vi "Main_No_OOP.vi"() -> ()   [LabVIEW 2020]
uses:
  <vilib>/vision/driver/NI_Vision_Acquisition_Software.lvlib
panel:
  in  "Stop":bool
  in  "Tipo de Cámara":enum32{"WebCam", "Simulada"}(tab)
  in  "Camaras Disponibles":u16(ring) items=["cam0", "cam1", "cam2", "cam3", "cam4"]
  in  "Aceptar":bool
  in  "Ruta IMG":path
  in  "Aceptar":bool
  out "Imagen":T1(plugin-control)
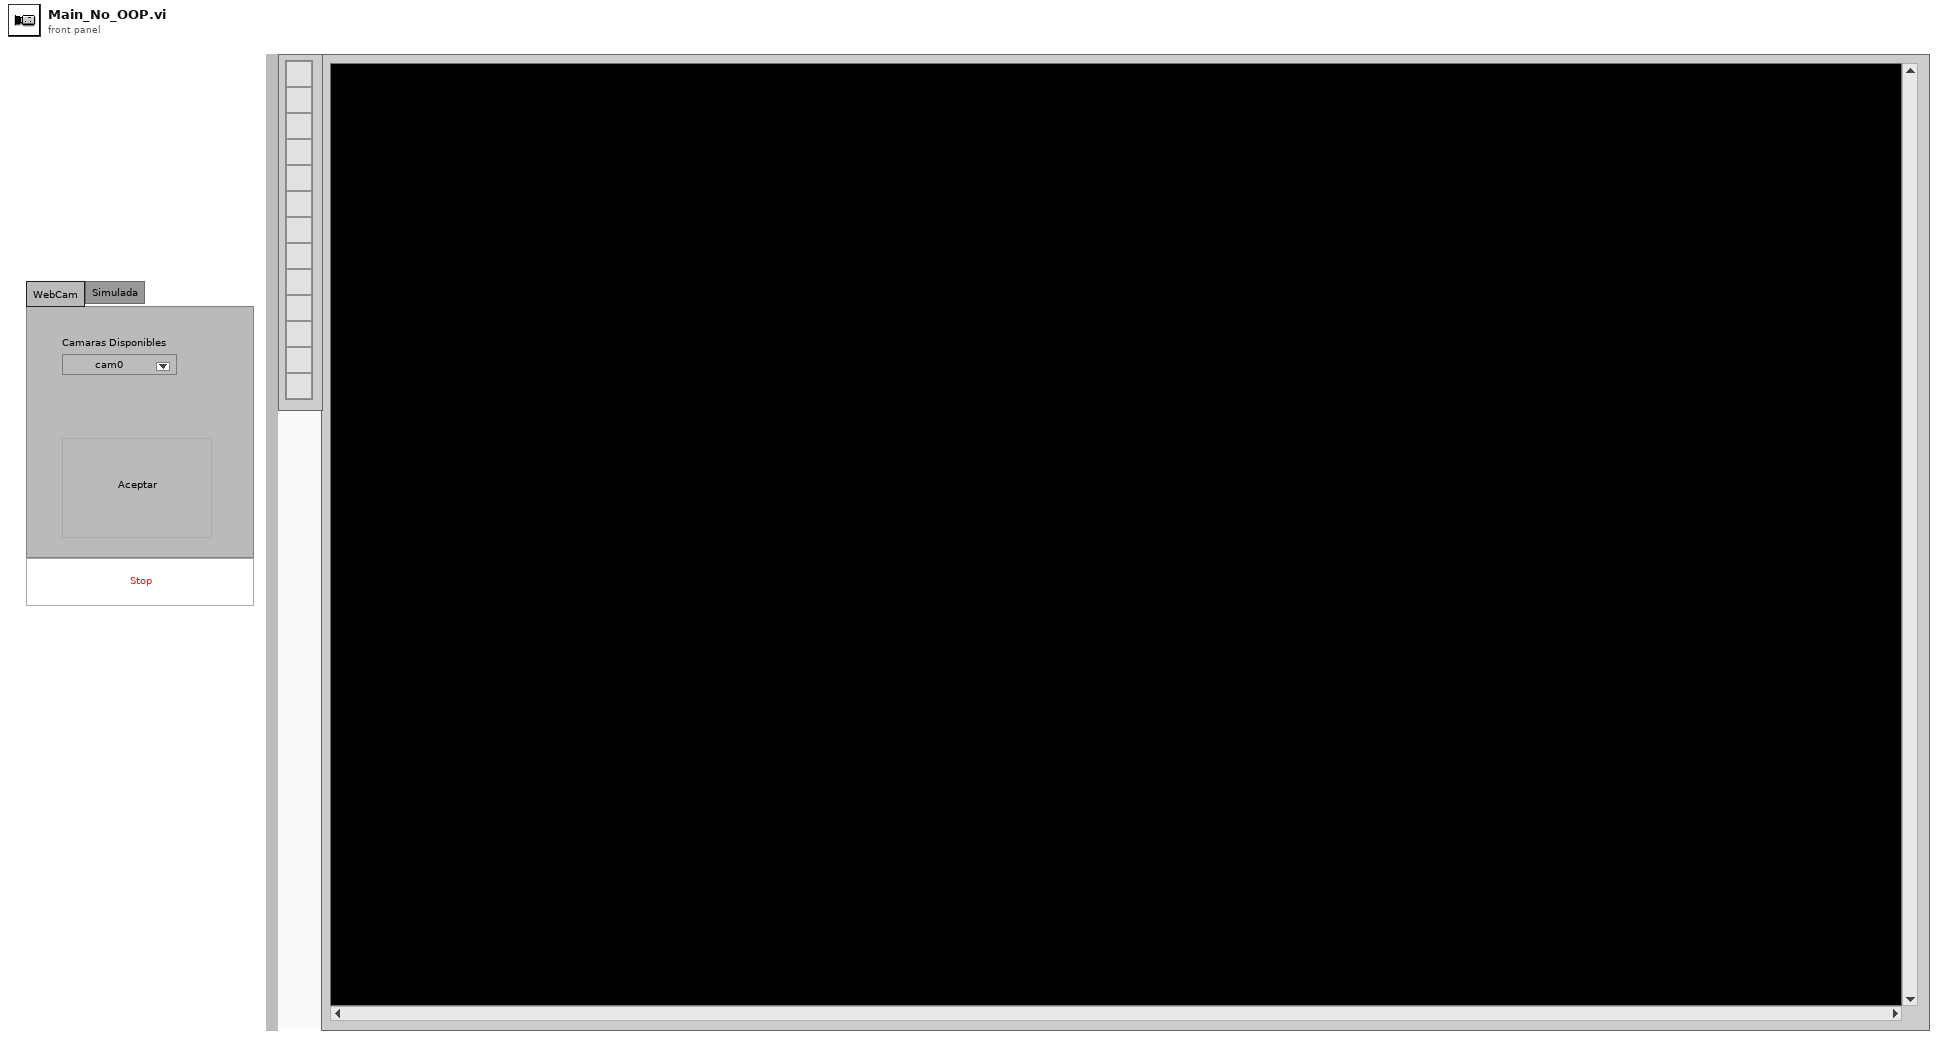
[diagram p1: front panel]
types:
  T1 = typedef "IMAQ Image.ctl" = refnum<image>
  T2 = typedef "Image Type" = u32
  T3 = cluster{"Type":u32, "Version":u32, "Flags":u32, "SerialNumberHigh":u32, "SerialNumberLow":u32, "BusType":u32, "InterfaceName":string, "VendorName":string, "ModelName":string, "CameraFileName":string, "CameraAttributeURL":string}[]
  T4 = typedef "IMAQdx.ctl" = refnum<k21>
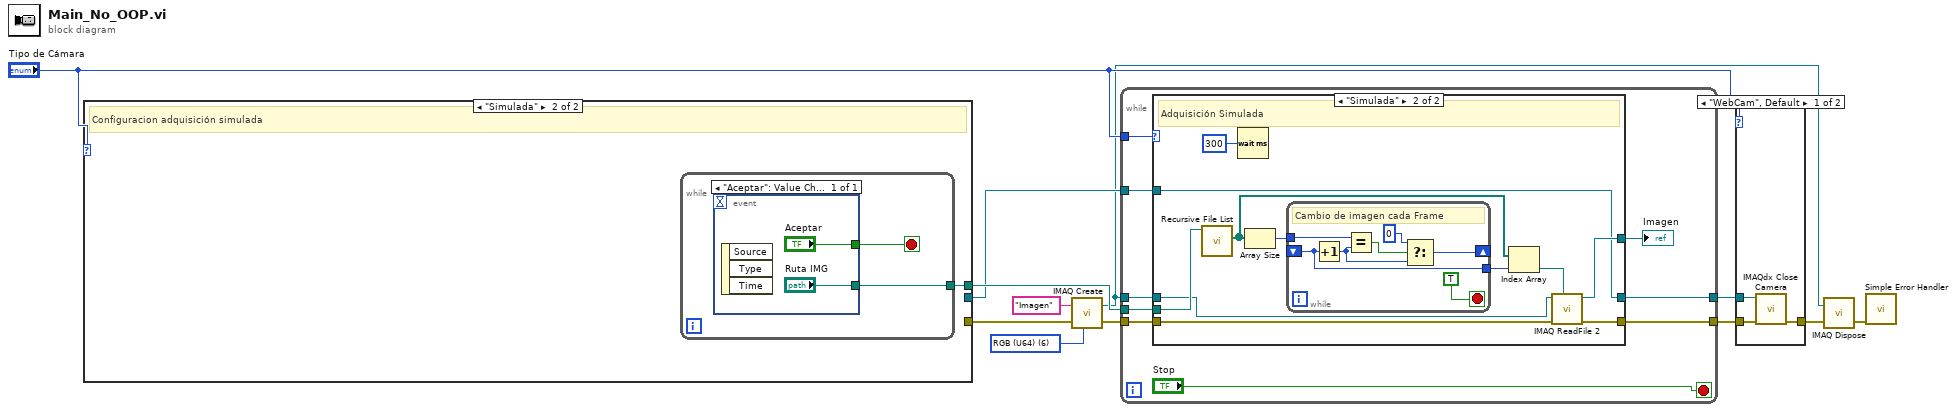
[diagram p0: block diagram]
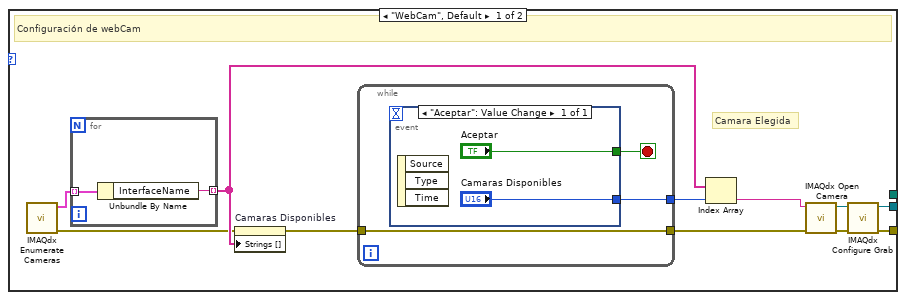
[diagram p2: hidden frame]
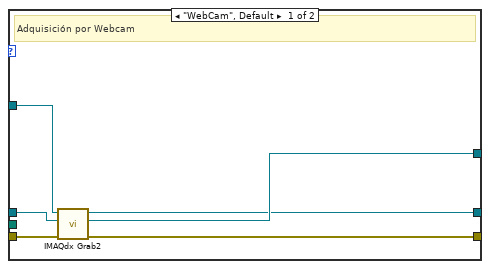
[diagram p4: hidden frame]
diagram:
  w8 = T2 6 items=["Grayscale (U8)", "Grayscale (I16)", "Grayscale (SGL)", "Complex (CSG)", "RGB (U32)", "HSL (U32)", "RGB (U64)", "Grayscale (U16)"] ("Image Type")
  n1 = case shown="\"Simulada\"" "Tipo de Cámara" {
    tunnel: [_ w31] -> w12
    tunnel: [w16 _] -> w11
    tunnel: [w15 _] -> w7
    frame "WebCam", Default {
      # "Camara Elegida"
      # "Configuración de webCam"
      n2 = call <vilib>:"IMAQdx Enumerate Cameras.vi"() -> ("error out"=w14:errorcluster, "Camera Information Array"=w23:T3)  [unwired: 10 in]
      n3 = for {
        tunnel: w23 -> [w30] mode=indexing
        tunnel: [w29] -> w21 mode=indexing
        n4 = Unbundle By Name(w30) -> ("InterfaceName"=w29:string)
      }
      n5 = property on="Camaras Disponibles" class="Ring (strict)"(error in=w14, "Strings []"=w21) -> (error out=w22:errorcluster)  [unwired: 1 in, 1 out]
      n6 = while {
        tunnel: w22 -> [w24]
        tunnel: [w25] -> w20
        tunnel: [w24] -> w13
        stop <- w26 stop-if-true
        n7 = event shown="[0] \"Aceptar\": Value Change" {
          selector: _ -> [_]
          dyn-events: _ -> [_]
          timeout: _ -> [_]
          tunnel: ["Aceptar"] -> w26
          tunnel: ["Camaras Disponibles"] -> w25
          event "Aceptar": Value Change {
            n8 = event-data() -> ()  [unwired: 1 in, 3 out]
          }
        }
      }
      n9 = Index Array(array=w21, index=w20) -> (element=w19:string)
      n10 = call <vilib>:"IMAQdx Open Camera.vi"("error in"=w13, "Session In"=w19) -> ("error out"=w17:errorcluster, "Session Out"=w18:T4)  [unwired: 8 in]
      n11 = call <vilib>:"IMAQdx Configure Grab.vi"("error in"=w17, "Session In"=w18) -> ("error out"=w16:errorcluster, "Session Out"=w15:T4)  [unwired: 8 in]
    }
    frame "Simulada" {
      # "Configuracion adquisición simulada"
      n12 = while {
        tunnel: [w32] -> w31
        stop <- w33 stop-if-true
        n13 = event shown="[0] \"Aceptar\": Value Change" {
          selector: _ -> [_]
          dyn-events: _ -> [_]
          timeout: _ -> [_]
          tunnel: ["Aceptar"] -> w33
          tunnel: ["Ruta IMG"] -> w32
          event "Aceptar": Value Change {
            n14 = event-data() -> ()  [unwired: 1 in, 3 out]
          }
        }
      }
    }
  }
  n15 = call "IMAQ Create"("Image Name"="Imagen", "Image Type"=w8, "error in (no error)"=w11) -> ("New Image"=w1:T1, "error out"=w10:errorcluster)  [unwired: 2 in]
  n16 = while {
    tunnel: w12 -> [w43]
    tunnel: "Tipo de Cámara" -> [w42]
    tunnel: w10 -> [w41]
    tunnel: w7 -> [w40]
    tunnel: w1 -> [w39]
    tunnel: [w38] -> w5
    tunnel: [w37] -> w4
    stop <- "Stop" stop-if-true
    n17 = case shown="\"Simulada\"" w42 {
      tunnel: [w47 w61] -> w44
      tunnel: w43 -> [_ w56]
      tunnel: w41 -> [w48 w55]
      tunnel: w40 -> [w49 w54]
      tunnel: w39 -> [w50 w51]
      tunnel: [w46 w54] -> w38
      tunnel: [w45 w53] -> w37
      frame "WebCam", Default {
        # "Adquisición por Webcam"
        n18 = call <vilib>:"IMAQdx Grab2.vi"("error in"=w48, "Image In"=w50, "Session In"=w49) -> ("error out"=w45:errorcluster, "Image Out"=w47:T1, "Session Out"=w46:T4)  [unwired: 5 in, 1 out]
      }
      frame "Simulada" {
        # "Adquisición Simulada"
        n19 = call <vilib>:"Recursive File List.vi"("Folder Path"=w56) -> ("All Files in Dir"=w59:path[])  [unwired: 6 in, 4 out]
        n20 = Wait (ms)(milliseconds to wait=u32 300) -> ()  [unwired: 1 out]
        n21 = Array Size(array=w59) -> (size(s)=w58:i32)
        n22 = while {
          tunnel: w58 -> [w68]
          shift-right: [w64] -> _
          shift-left: _ -> [w62]
          tunnel: [w62] -> w57
          stop <- TRUE stop-if-true
          # "Cambio de imagen cada Frame"
          n23 = Increment(x=w62) -> (x+1=w66:i32)
          n24 = Equal?(x=w68, y=w66) -> (x = y?=w67:bool)
          n25 = Select(t=0, s=w67, f=w66) -> (s? t:f=w64:i32)
        }
        n26 = Index Array(array=w59, index=w57) -> (element=w60:path)
        n27 = call "IMAQ ReadFile 2"("File Path"=w60, "error in (no error)"=w55, "Image"=w51) -> ("error out"=w53:errorcluster, "Image Out"=w61:T1)  [unwired: 4 in, 3 out]
      }
    }
    "Imagen" <- w44
  }
  n28 = case shown="\"WebCam\", Default" "Tipo de Cámara" {
    tunnel: w5 -> [w71 _]
    tunnel: w4 -> [w70 w72]
    tunnel: [w69 w72] -> w3
    frame "WebCam", Default {
      n29 = call <vilib>:"IMAQdx Close Camera.vi"("error in"=w70, "Session In"=w71) -> ("error out"=w69:errorcluster)  [unwired: 9 in]
    }
    frame "Simulada" {
    }
  }
  n30 = call "IMAQ Dispose"("Image"=w1, "error in (no error)"=w3) -> ("error out"=w2:errorcluster)  [unwired: 4 in]
  n31 = call <vilib>:"Simple Error Handler.vi"("error in (no error)"=w2) -> ()  [unwired: 4 in, 5 out]
